vi "PersistantClassData.vi"() -> ()   [LabVIEW 2019, in "GlobalTestData.lvclass"]
uses:
  GlobalTestData.lvclass
panel:
  in  "GlobalTestData":refnum<class "GlobalTestData.lvclass">
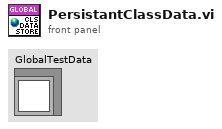
[diagram p1: front panel]
diagram:
